vi "lowpass.vi"(11 "In_k":dbl) -> ()   [LabVIEW 2019]
panel:
  out "filter output":dbl
  in  "Ts":dbl
  in  "Tf":dbl
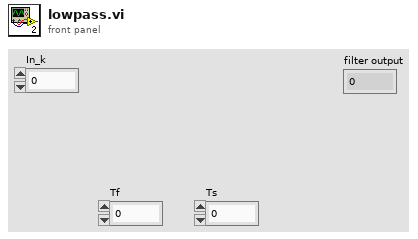
[diagram p1: front panel]
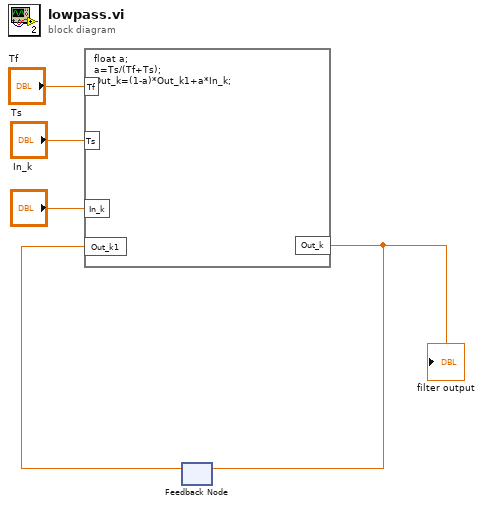
[diagram p0: block diagram]
diagram:
  n1 = feedback #1() -> (w1:dbl)  [unwired: 1 in]
  n2 = formula code="float a;\na=Ts/(Tf+Ts);\nOut_k=(1-a)*Out_k1+a*In_k;"("Tf"="Tf", "Ts"="Ts", "In_k"="In_k", "Out_k1"=w1) -> ("Out_k"=w2:dbl)
  "filter output" <- w2
  n3 = feedback-in #1(w2) -> ()
